vi "Get Wheel Type.vi"(8 "error in (no error)":errorcluster, 11 "omni wheel in":refnum<class "NI_Robotics_Omnidirectional Wheel.lvclass">) -> (0 "error out":errorcluster, 2 "wheel type":string, 3 "omni wheel out":refnum<class "NI_Robotics_Omnidirectional Wheel.lvclass">)   [LabVIEW 2017, in "NI_Robotics_Omnidirectional Wheel.lvclass"]
uses:
  <vilib>/robotics/Steering/Omnidirectional Wheel/NI_Robotics_Omnidirectional Wheel.lvclass
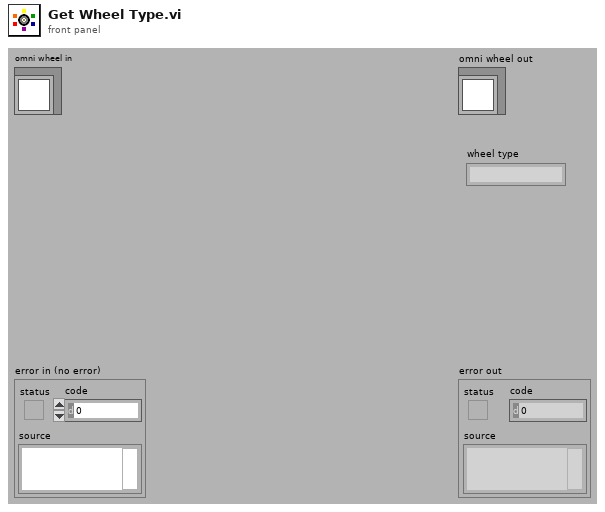
[diagram p1: front panel]
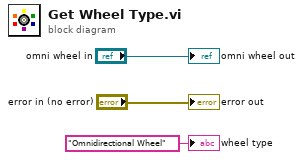
[diagram p0: block diagram]
diagram:
  "error out" <- "error in (no error)"
  "omni wheel out" <- "omni wheel in"
  "wheel type" <- "Omnidirectional Wheel" ("wheel type")
